vi "BotStatus.vi"() -> ()   [LabVIEW 2012]
panel:
  in  "Calculated zAvit":dbl
  in  "Axis X":dbl
  in  "Whole robot centering":bool
  in  "center on target":bool
  in  "View ground":bool
  in  "Stop auto camera movment":bool
  in  "axis 3 camera controller joystick":dbl
  in  "Y axis camera controller joystick":dbl
  in  "Ready to Fire":bool
  in  "RPM Set":bool
  in  "Throttle attack 3":dbl
  in  "Throttle 3D pro":dbl
  in  "Disable Stack":bool
  in  "Canenet Right":dbl
  in  "Camera Servo Y":dbl
  in  "Camera Servo X":dbl
  in  "Feeder":dbl
  in  "Canenet Left":dbl
  in  "zAvit":dbl
  in  "Cannon":dbl
  in  "Transfer":dbl
  in  "Flipper":dbl
  in  "Conveyer Belt":dbl
  in  "Roller":dbl
  in  "Camera Centered":bool
  in  "overrides":dbl[](array[numeric])
  in  "Cannon LS":T1
  in  "Frisbee in Stack Counter":i32
  in  "Collect from Feeder?":bool
  in  "Target Info":T2
  in  "Empty Stack":bool
  in  "Distance [m]":dbl
  in  "Climbing":bool
  in  "Cannon Position(deg)":dbl
  in  "Frisbee States":T3
  # "Cannon"
  # "From end of cannon to center of target"
  # "InCannon"
  # "InFlipper"
  # "FlipperAtPlace"
  # "Middle"
  # "Bottom"
  # "UPDATES VALUES IN Periodic Tasks.vi"
  # "Feeder Angle"
  # "Flipper Angle"
  # "Cannon Angle"
  # "90"
  # "90"
  # "90"
  # "131"
  # "170"
  # "170"
  # "0"
  # "48.6 => 49"
  # "0"
  # "-min angle"
  # "0"
  # "\"Cannon Position(deg)\""
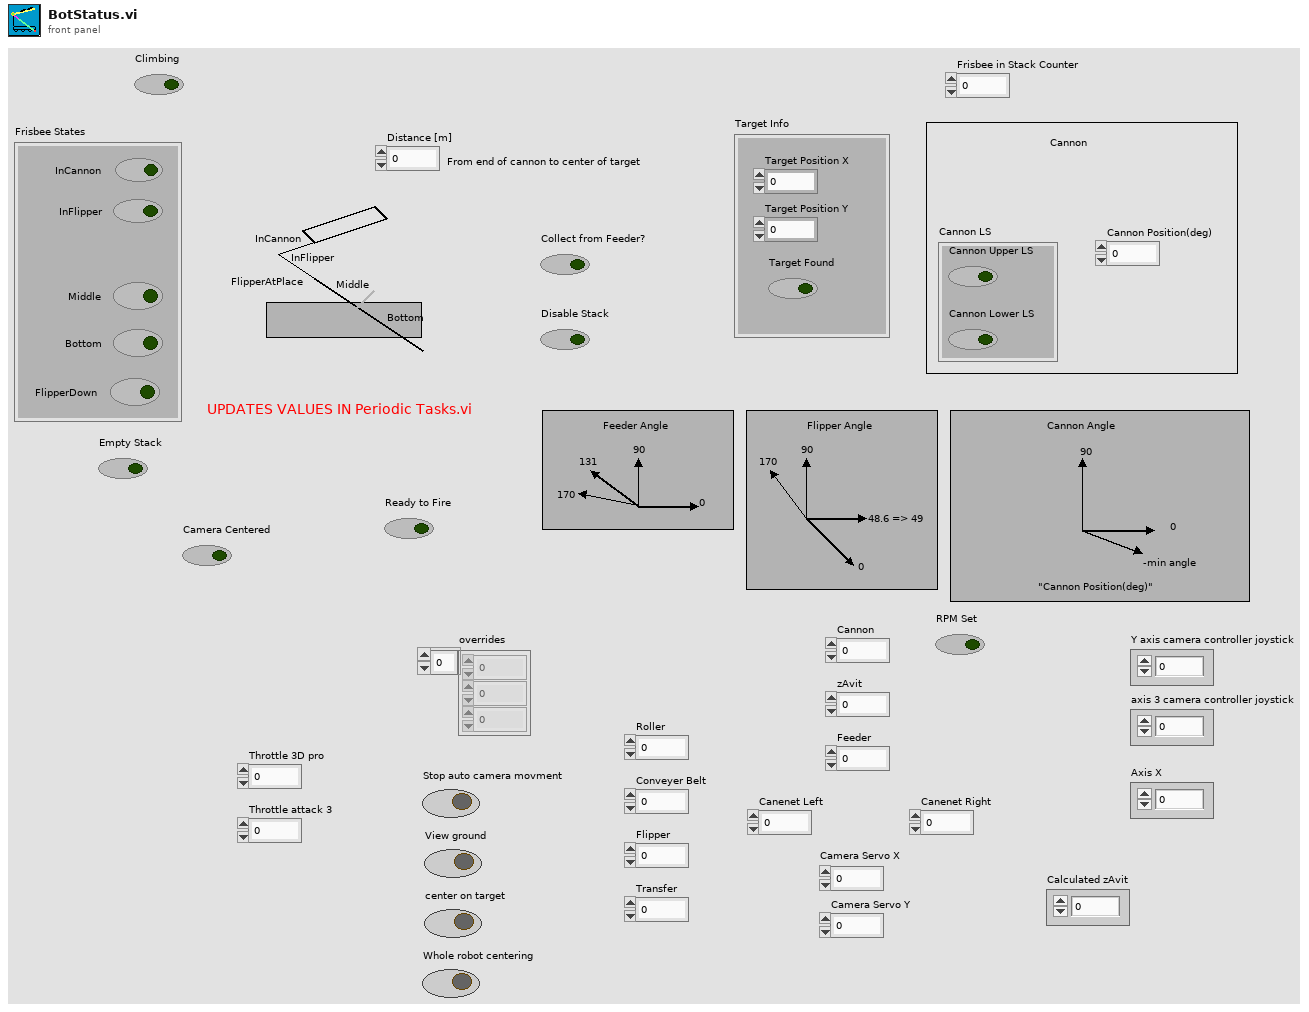
[diagram p1: front panel]
types:
  T1 = cluster{"Cannon Upper LS":bool, "Cannon Lower LS":bool}
  T2 = cluster{"Target Position X":dbl, "Target Position Y":dbl, "Target Found":bool}
  T3 = cluster{"Middle":bool, "InCannon":bool, "InFlipper":bool, "Bottom":bool, "FlipperDown":bool}
diagram:
